vi "Class.SaveCtrls.Init.vi"(7 "Module Name":string, 8 "error in (no error)":errorcluster, 9 "Ctrl Array":refnum<vi>[](array[refnum]), 10 "Module Data Dir":path, 11 "Save Control States in":refnum<class "Class.SaveCtrls.lvclass">) -> (0 "error out":errorcluster, 3 "Save Control States out":refnum<class "Class.SaveCtrls.lvclass">)   [LabVIEW 2024, in "EQMF.lvlib" / "Config Utils.lvlib" / "Class.SaveCtrls.lvclass"]
uses:
  Class.SaveCtrls.lvclass
  Class.SaveCtrls.lvclass/Class.SaveCtrls.ctl
  <vilib>/Utility/sysdir.llb/System Directory Type.ctl
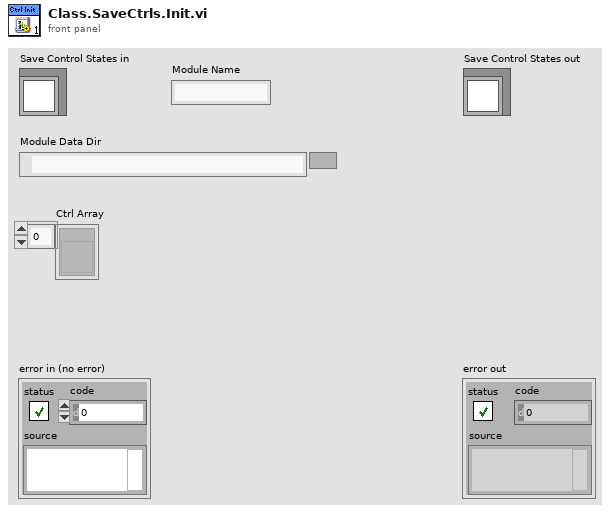
[diagram p1: front panel]
types:
  T1 = typedef "System Directory Type.ctl" = i32
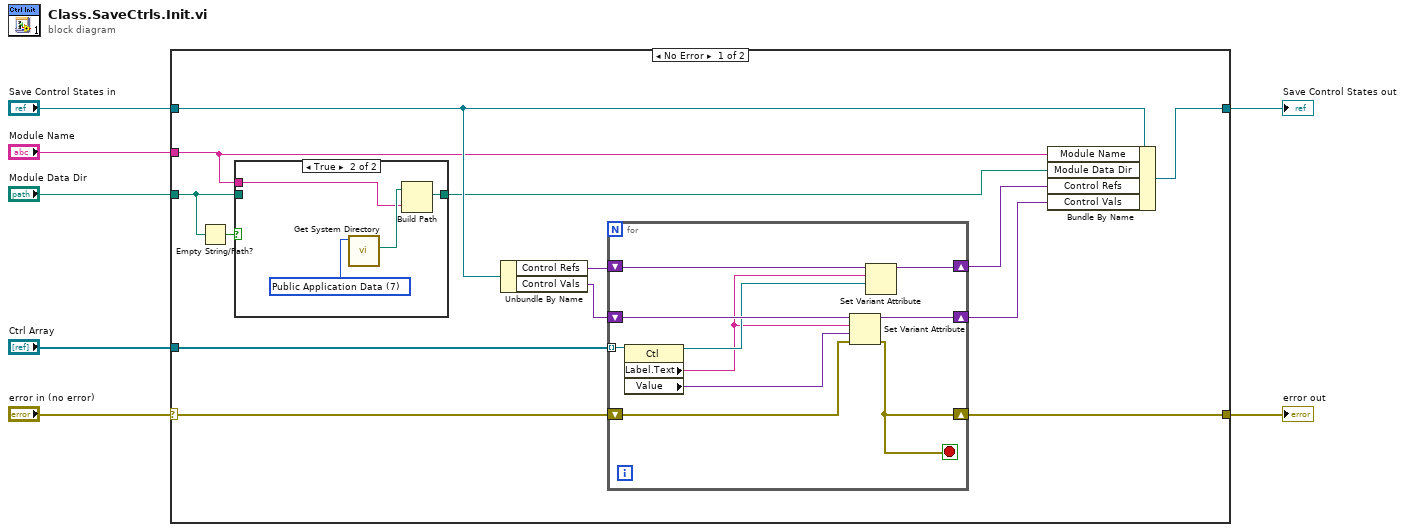
[diagram p0: block diagram]
diagram:
  n1 = case shown="No Error" "error in (no error)" {
    selector: "error in (no error)" -> [w16 w37]
    tunnel: [w17 w37] -> w6
    tunnel: [w12 w36] -> w4
    tunnel: "Save Control States in" -> [w13 w36]
    tunnel: "Module Name" -> [w8 _]
    tunnel: "Module Data Dir" -> [w10 _]
    tunnel: "Ctrl Array" -> [w18 _]
    frame No Error {
      n2 = Empty String/Path?(string/path=w10) -> (empty?=w11:bool)
      n3 = case shown="True" w11 {
        tunnel: w10 -> [w21 _]
        tunnel: [w21 w24] -> w9
        tunnel: w8 -> [_ w22]
        frame False {
        }
        frame True {
          w25 = T1 7 items=["User Home"=0, "User Desktop"=1, "User Documents"=2, "User Application Data"=3, "User Preferences"=4, "User Temporary"=5, "Public Documents"=6, "Public Application Data"=7, "Public Preferences"=8, "Public Cache"=13, "System Core Libraries"=9, "System Installed Libraries"=10, "Application Files"=11, "Boot Volume Root"=12] ("system directory type")
          n4 = call <vilib>:"Get System Directory.vi"("system directory type"=w25) -> ("system directory"=w23:path)  [unwired: 10 in]
          n5 = Build Path(base path=w23, name or relative path=w22) -> (appended path=w24:path)
        }
      }
      n6 = Unbundle By Name(w13) -> ("Control Refs"=w20:variant, "Control Vals"=w19:variant)
      n7 = for {
        shift-right: [w31] -> w17
        shift-left: w16 -> [w33]
        tunnel: w18 -> [w32] mode=indexing
        shift-right: [w34] -> w14
        shift-left: w19 -> [w35]
        shift-right: [w27] -> w15
        shift-left: w20 -> [w30]
        stop <- w31 stop-if-true
        n8 = property class="Ctl"(reference=w32) -> (reference out=w29:refnum<vi>, "Label.Text"=w26:string, "Value"=w28:variant)  [unwired: 1 in, 1 out]
        n9 = Set Variant Attribute(Variant=w35, name=w26, value=w28, error in=w33) -> (Variant out=w34:variant, error out=w31:errorcluster)  [unwired: 1 out]
        n10 = Set Variant Attribute(Variant=w30, name=w26, value=w29) -> (Variant out=w27:variant)  [unwired: 1 in, 2 out]
      }
      n11 = Bundle By Name(cluster=w13, "Module Name"=w8, "Module Data Dir"=w9, "Control Refs"=w15, "Control Vals"=w14) -> (w12:refnum<class "Class.SaveCtrls.lvclass">)
    }
    frame Error {
    }
  }
  "error out" <- w6
  "Save Control States out" <- w4
